vi "Calibrate P2t.vi"(4 "Calibration Grid File Path":path=path "C:/Users/serce/Desktop/Smart Vision System Testbench/Grid Calibration.png", 5 "Error In":errorcluster, 8 "Image In":T1) -> (0 "Error Out":errorcluster, 3 "Image Out":T1)   [LabVIEW 2020]
uses:
  <vilib>/vision/Image Controls.llb/IMAQ Image.ctl
  <vilib>/vision/NI_Vision_Development_Module.lvlib
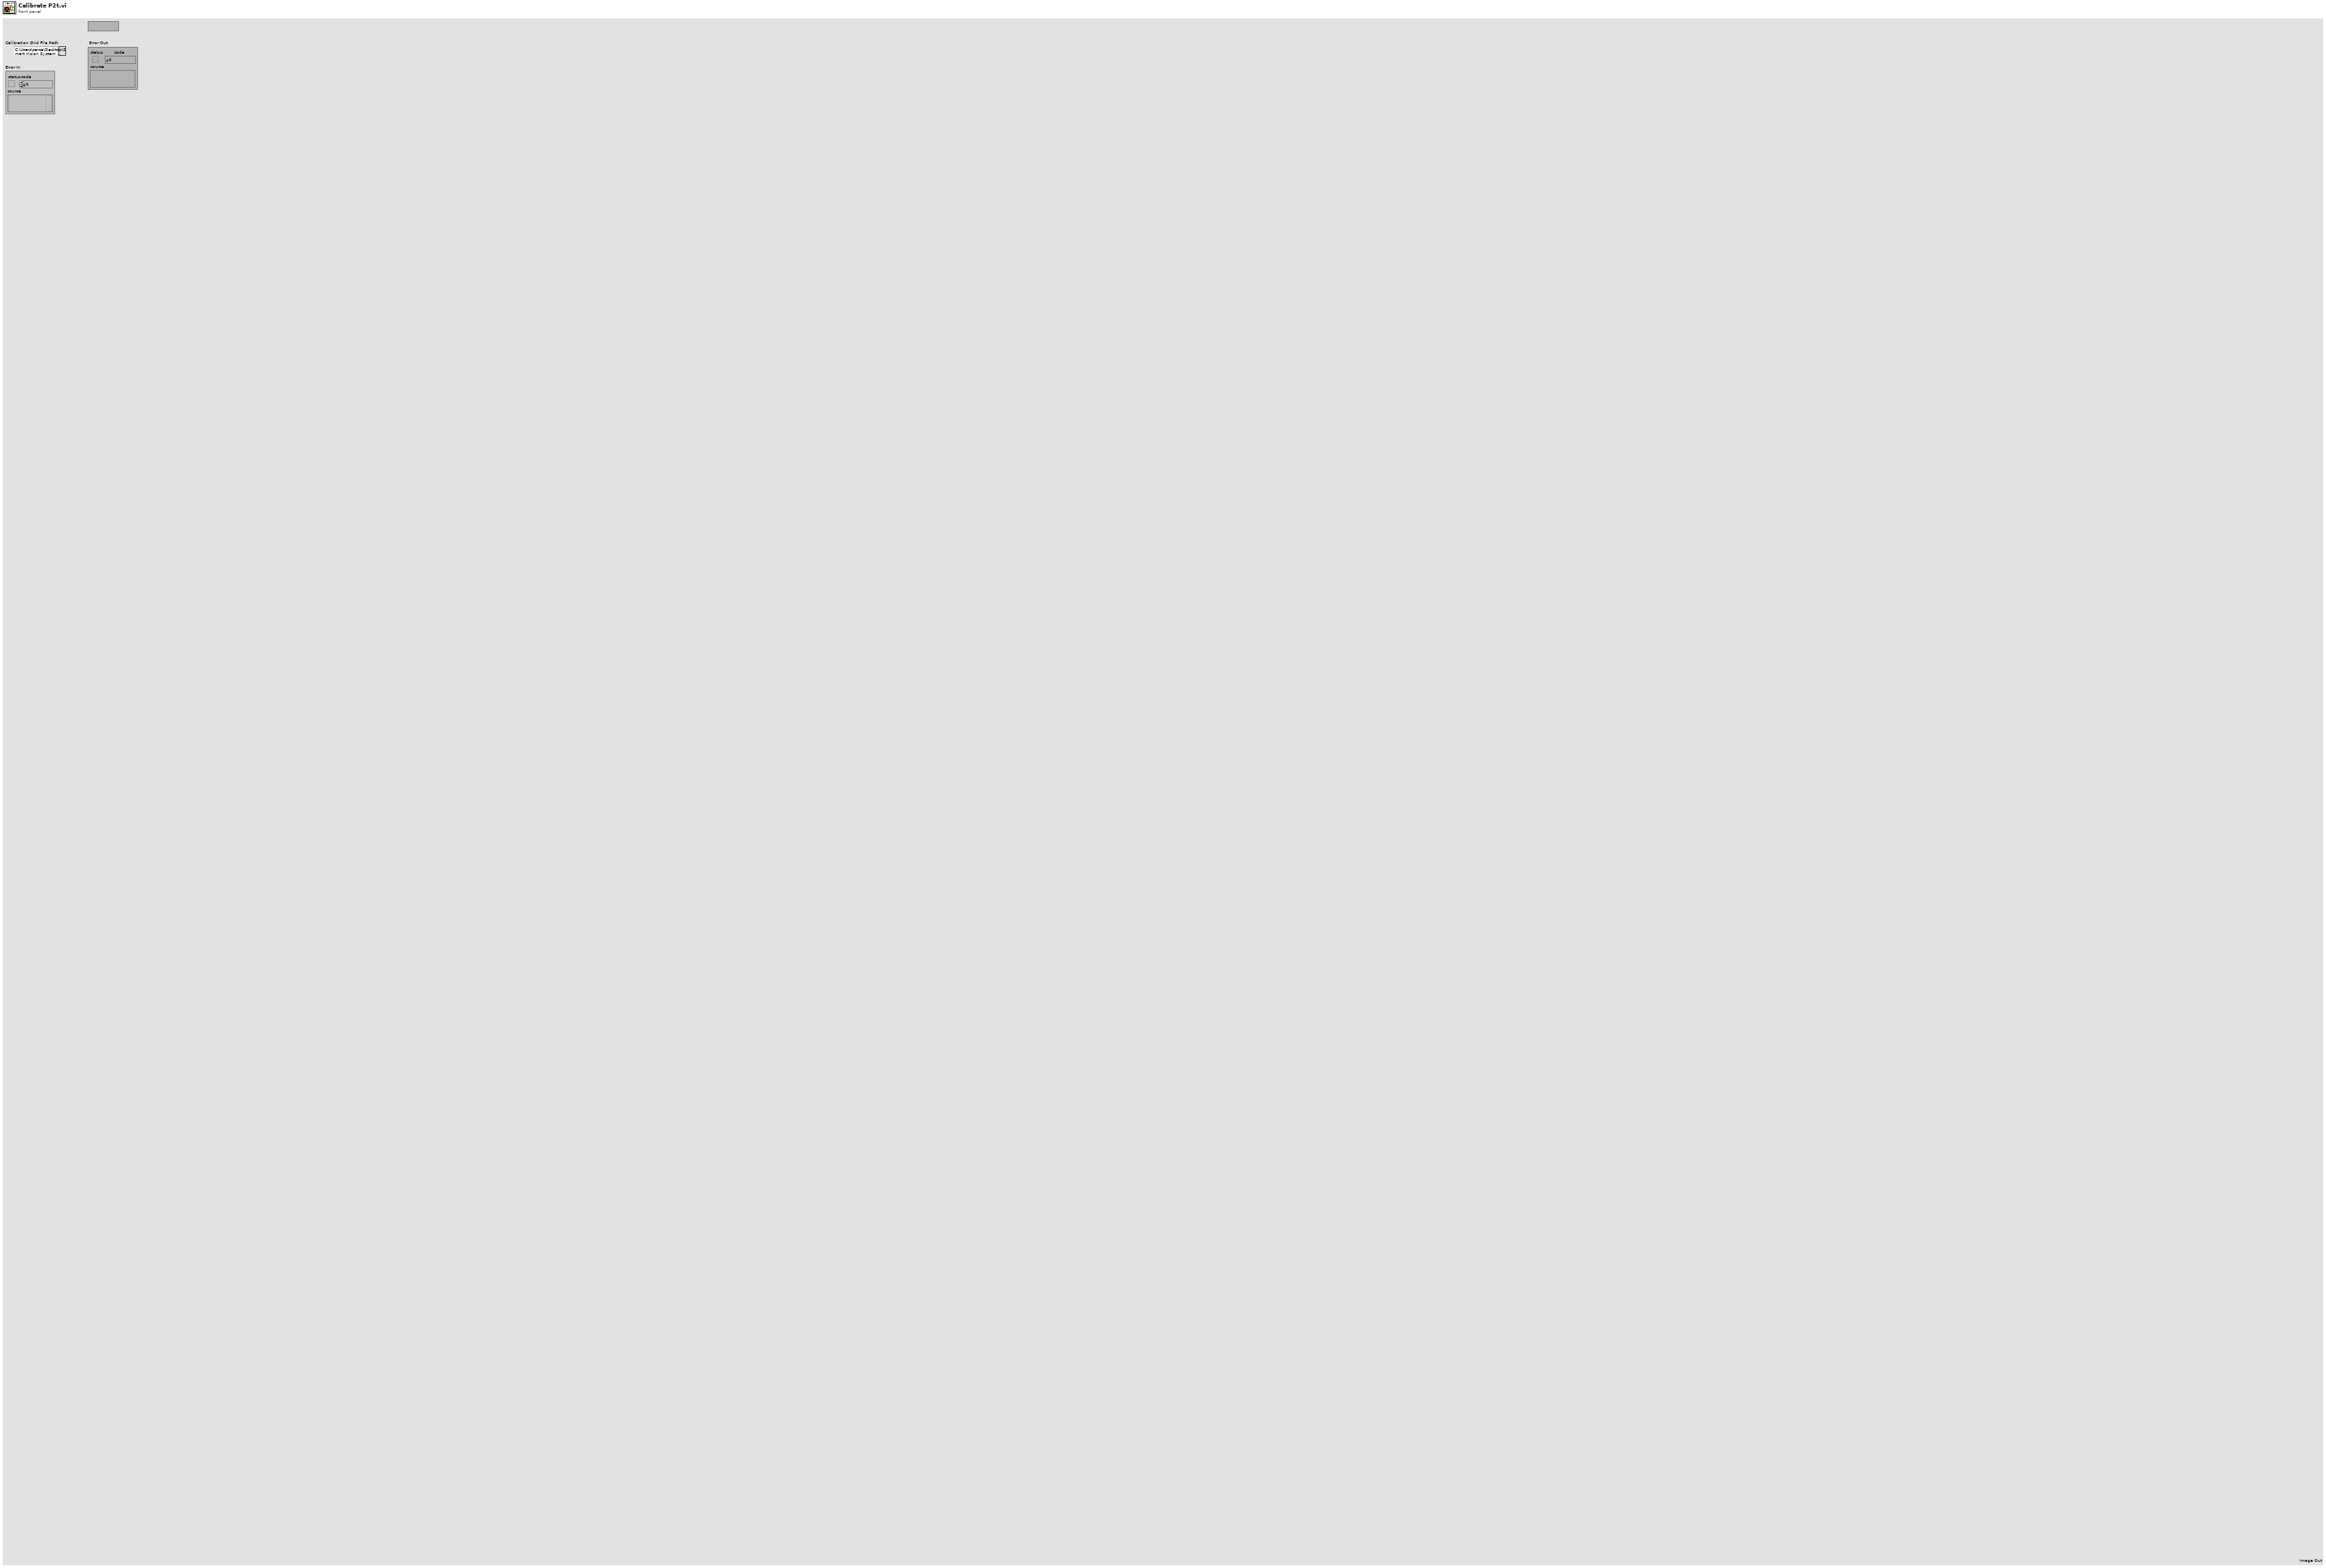
[diagram p1: front panel]
types:
  T1 = typedef "IMAQ Image.ctl" = refnum<image>
  T2 = cluster{"Origin Pixel":cluster{"X":sgl, "Y":sgl}, "X Axis Pixel":cluster{"X":sgl, "Y":sgl}, "Axis Reference":u32}
  T3 = cluster{"Brightness":sgl, "Contrast":sgl, "Gamma":sgl}
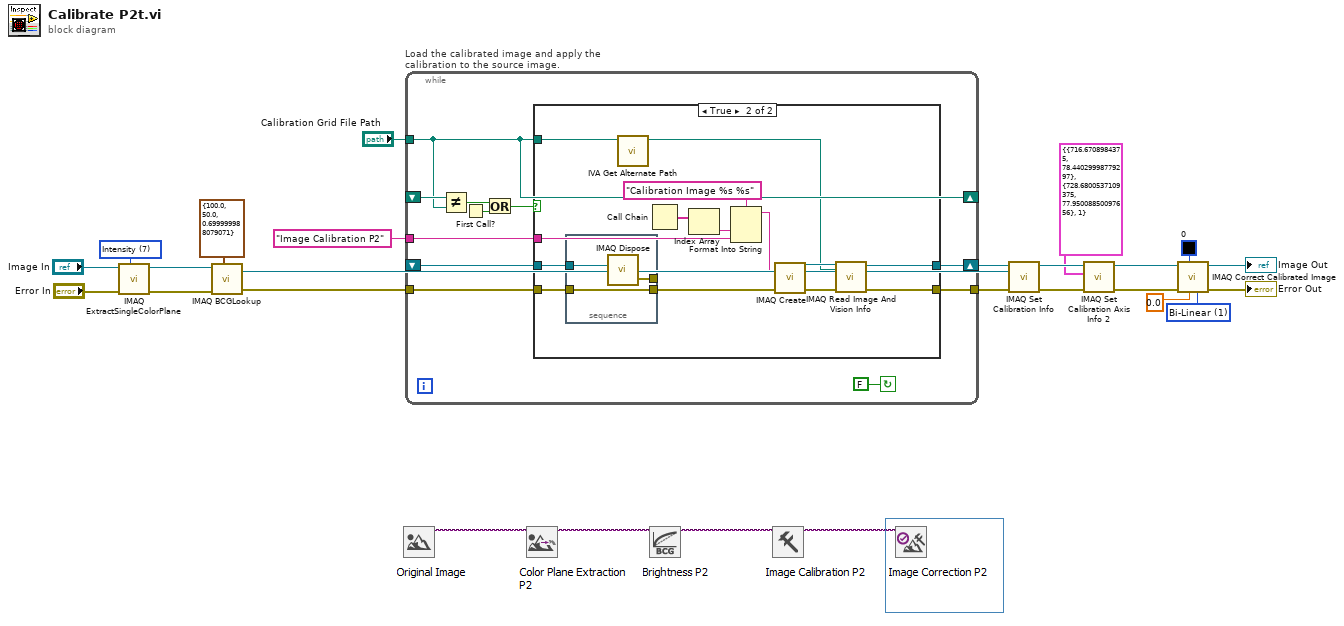
[diagram p0: block diagram]
diagram:
  w7 = u32 1 items=["Zero Order", "Bi-Linear", "Quadratic", "Cubic Spline"] ("Interpolation Type")
  w22 = 7 items=["Red", "Green", "Blue", "Hue", "Saturation", "Luminance", "Value", "Intensity"] ("Color Plane")
  n1 = call "IMAQ ExtractSingleColorPlane"("Color Plane"=w22, "error in (no error)"="Error In", "Image Src"="Image In") -> ("error out"=w18:errorcluster, "Image Dst Out"=w19:T1)  [unwired: 1 in, 6 out]
  n2 = call "IMAQ BCGLookup"("Image Src"=w19, "BCG Values"=T3 {"Brightness"=100.0, "Contrast"=50.0, "Gamma"=0.7}, "error in (no error)"=w18) -> ("Image Dst Out"=w12:T1, "error out"=w16:errorcluster)  [unwired: 2 in, 2 out]
  n3 = while "Load the calibrated image and apply the calibration to the source image." {
    shift-right: [w33] -> w14
    shift-left: _ -> [w32]
    tunnel: [w30] -> w13
    tunnel: w16 -> [w29]
    tunnel: "Calibration Grid File Path" -> [w26]
    tunnel: "Image Calibration P2" ("Step Name") -> [w28]
    shift-right: [w26] -> _
    shift-left: _ -> [w27]
    stop <- FALSE continue-if-true
    n4 = Not Equal?(x=w27, y=w26) -> (x != y?=w24:bool)
    n5 = First Call?() -> (First Call?: T/F=w25:bool)
    n6 = Or(x=w24, y=w25) -> (x .or. y?=w23:bool)
    n7 = case shown="True" w23 {
      tunnel: [w35 w47] -> w33
      tunnel: w32 -> [w35 w39]
      tunnel: [w34 w44] -> w30
      tunnel: w29 -> [w34 w40]
      tunnel: w26 -> [_ w37]
      tunnel: w28 -> [_ w41]
      frame False {
      }
      frame True {
        n8 = stacked-sequence {
          tunnel: w40 -> [w51]
          tunnel: w39 -> [w52]
          tunnel: [w51] -> w38
          tunnel: [w50] -> _
          frame #0 {
            n9 = call "IMAQ Dispose"("Image"=w52) -> ("error out"=w50:errorcluster)  [unwired: 2 in, 3 out]
          }
        }
        n10 = call <vilib>:"IVA Get Alternate Path.vi"("Path In"=w37) -> ("Path Out"=w36:path)  [unwired: 10 out]
        n11 = Call Chain() -> (call chain=w43:string[])
        n12 = Index Array(array=w43) -> (element=w42:string)  [unwired: 1 in]
        n13 = Format Into String(format string="Calibration Image %s %s" ("Image Name"), w42, w41) -> (resulting string=w49:string)  [unwired: 2 in, 1 out]
        n14 = call "IMAQ Create"("Image Name"=w49, "error in (no error)"=w38) -> ("New Image"=w46:T1, "error out"=w45:errorcluster)  [unwired: 2 in, 1 out]
        n15 = call "IMAQ Read Image And Vision Info"("File Path"=w36, "error in (no error)"=w45, "Image"=w46) -> ("error out"=w44:errorcluster, "Image Out"=w47:T1)  [unwired: 1 in, 6 out]
      }
    }
  }
  n16 = call "IMAQ Set Calibration Info"("error in (no error)"=w13, "Image Dst"=w12, "Image Src"=w14) -> ("error out"=w9:errorcluster, "Calibrated Image"=w10:T1)  [unwired: 1 in, 6 out]
  n17 = call-poly "IMAQ Set Calibration Axis Info 2"("error in (no error)"=w9, "Calibration Axis Info"=T2 {"Origin Pixel"={"X"=716.6709, "Y"=78.4403}, "X Axis Pixel"={"X"=728.68005, "Y"=77.95009}, "Axis Reference"=1}, "Calibration Template Image In"=w10) -> ("error out"=w3:errorcluster, "Calibration Template Image Out"=w4:T1)  [unwired: 7 out]
  n18 = call "IMAQ Correct Calibrated Image"("Interpolation Type"=w7, "Replace Value"=sgl 0.0, "Color Replace Value"=u32 0, "error in (no error)"=w3, "Image Src"=w4) -> ("error out"=→"Error Out":errorcluster, "Corrected Image"=→"Image Out":T1)  [unwired: 2 in, 3 out]
